vi "string matching 8.vi"() -> ()   [LabVIEW 2025]
panel:
  out "String 3":string
  out "String 2":string
  in  "String":string
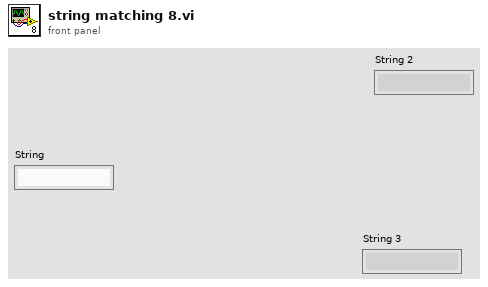
[diagram p1: front panel]
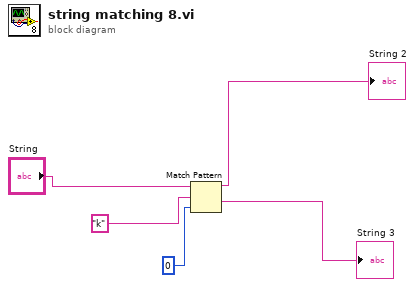
[diagram p0: block diagram]
diagram:
  n1 = Match Pattern(string="String", regular expression="k", offset (0)=0) -> (before substring=→"String 2":string, after substring=→"String 3":string)  [unwired: 2 out]
